vi "Save-As-Default (SubVI).vi"(0 "Current VI's Path":path, 2 "Load Settings":bool, 4 "Save Settings":bool, 9 "Save and Exit":bool) -> (19 "Save as Default Error":errorcluster)   [LabVIEW 2009]
panel:
  # "Save As Defaults (SubVI) - Created by Blake Otting - October 2007\nUpdated 4/7/2010"
  # "Connect As Shown \nin Main Program VI"
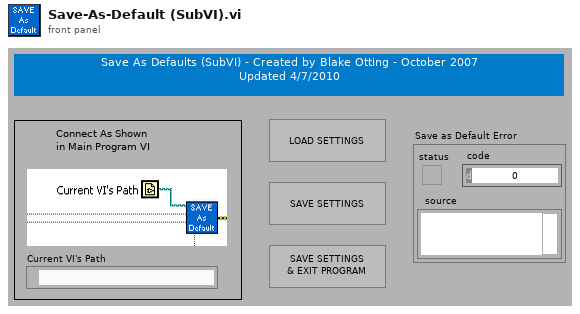
[diagram p1: front panel]
types:
  T1 = enum16{"open", "replace", "create", "open or create", "replace or create", "replace or create with confirmation"}
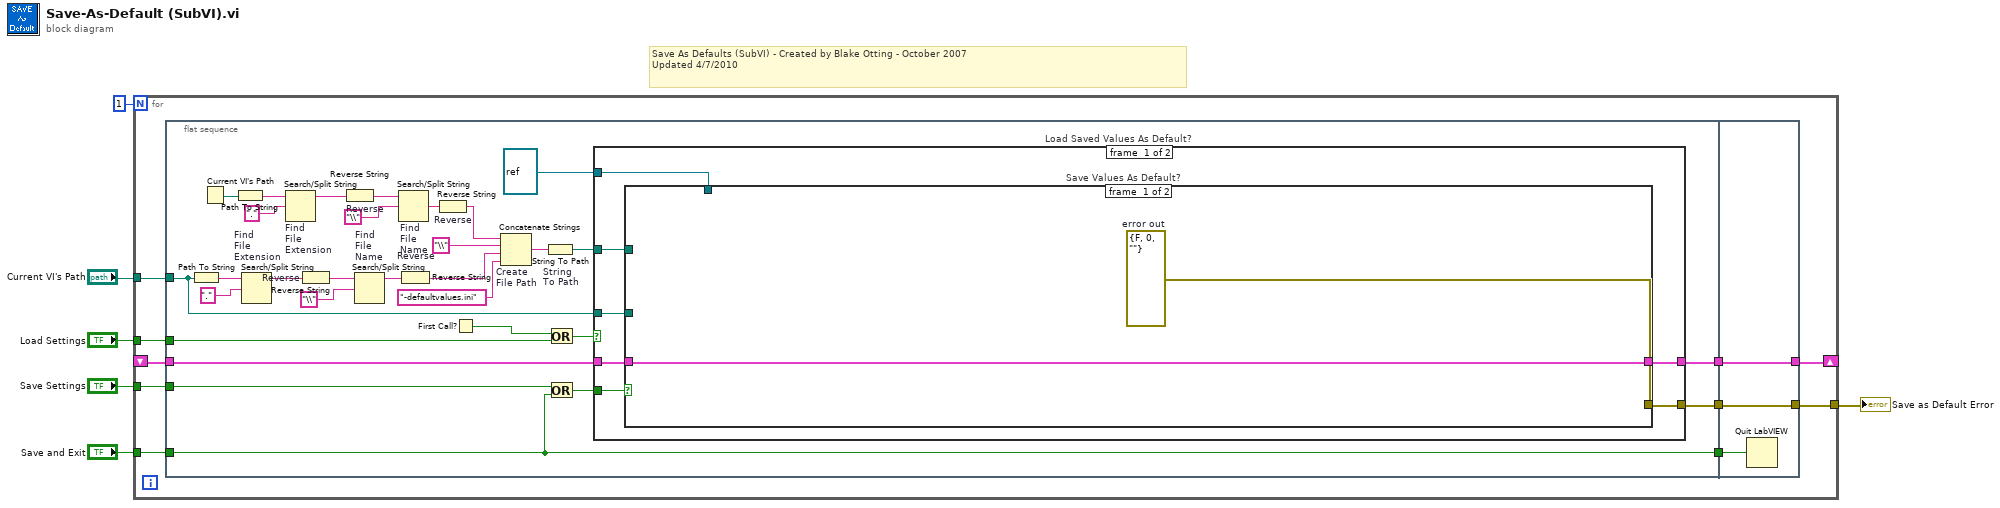
[diagram p0: block diagram]
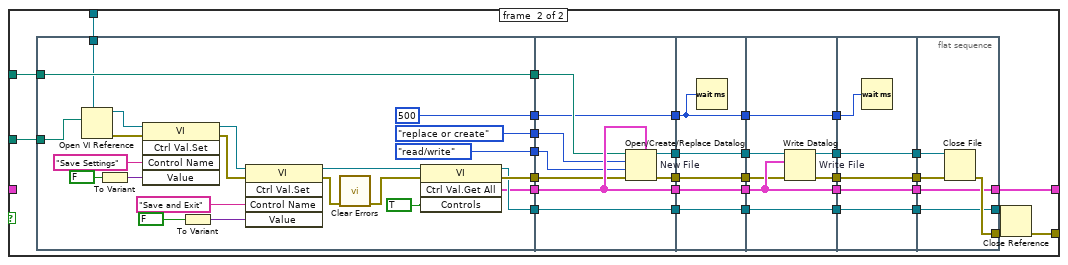
[diagram p2: hidden frame]
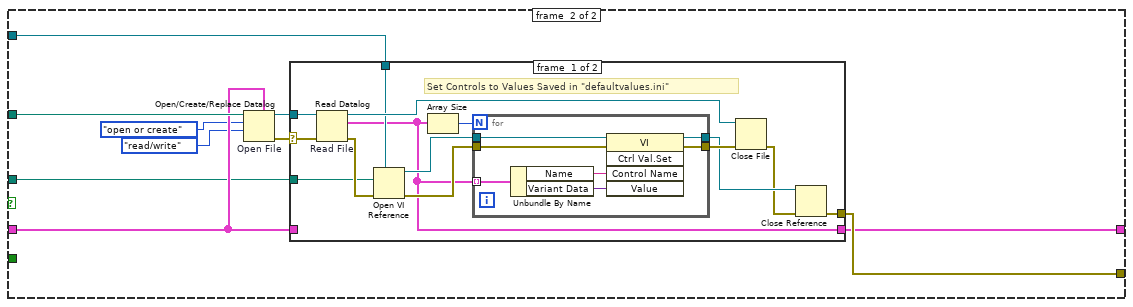
[diagram p3: hidden frame]
diagram:
  # "Save As Defaults (SubVI) - Created by Blake Otting - October 2007\nUpdated 4/7/2010"
  n1 = for {
    N: 1 -> [_]
    tunnel: "Current VI's Path" -> [w15]
    shift-right: [w16] -> _
    shift-left: _ -> [w14]
    tunnel: [w13] -> w1
    tunnel: "Save and Exit" -> [w8]
    tunnel: "Load Settings" -> [w7]
    tunnel: "Save Settings" -> [w9]
    n2 = flat-sequence {
      tunnel: [w45] -> w12
      tunnel: [w42] -> w11
      tunnel: [w41] -> w10
      tunnel: w7 -> [w39]
      tunnel: w8 -> [w41]
      tunnel: w9 -> [w40]
      tunnel: w15 -> [w38]
      tunnel: w14 -> [w46]
      tunnel: [w177] -> w13
      tunnel: [w178] -> w16
      tunnel: w12 -> [w178]
      tunnel: w11 -> [w177]
      tunnel: w10 -> [w176]
      frame #0 {
        n3 = Path To String(path=w38) -> (string=w25:string)
        n4 = Current VI's Path() -> (path=w20:path)
        n5 = Path To String(path=w20) -> (string=w32:string)
        n6 = Search/Split String "Find\nFile \nExtension"(string=w25, search string/char (-)=".") -> (substring before match=w22:string)  [unwired: 1 in, 2 out]
        n7 = Search/Split String "Find\nFile \nExtension"(string=w32, search string/char (-)=".") -> (substring before match=w31:string)  [unwired: 1 in, 2 out]
        n8 = Reverse String "Reverse"(1:w22) -> (0:w24:string)
        n9 = Reverse String "Reverse"(1:w31) -> (0:w30:string)
        n10 = Search/Split String "Find\nFile \nName"(string=w24, search string/char (-)="\\") -> (substring before match=w21:string)  [unwired: 1 in, 2 out]
        n11 = Search/Split String "Find\nFile \nName"(string=w30, search string/char (-)="\\") -> (match + rest of string=w28:string)  [unwired: 1 in, 2 out]
        n12 = Reverse String "Reverse"(1:w21) -> (0:w18:string)
        n13 = Reverse String "Reverse"(1:w28) -> (0:w27:string)
        n14 = First Call?() -> (First Call?: T/F=w34:bool)
        n15 = Concatenate Strings "Create\nFile Path"(w27, "\\", w18, "-defaultvalues.ini") -> (w36:string)
        n16 = String To Path "String\nTo Path"(string=w36) -> (path=w37:path)
        n17 = Or(x=w34, y=w39) -> (x .or. y?=w44:bool)
        n18 = Or(x=w40, y=w41) -> (x .or. y?=w43:bool)
        n19 = case "Load Saved Values As Default?" shown="False" w44 {
          tunnel: [w53 w152] -> w42
          tunnel: w37 -> [w52 w150]
          tunnel: w43 -> [w51 _]
          tunnel: w46 -> [w50 w149]
          tunnel: [w47 w151] -> w45
          tunnel: w38 -> [w49 w147]
          tunnel: refnum<vi> refnum ("Application Reference Input 2") -> [w48 w148]
          frame #0 {
            n20 = case "Save Values As Default?" shown="True" w51 {
              tunnel: [w54 w88] -> w53
              tunnel: w52 -> [_ w87]
              tunnel: [w55 w86] -> w47
              tunnel: w50 -> [w55 _]
              tunnel: w49 -> [_ w56]
              tunnel: w48 -> [_ w57]
              frame #0 {
                w54 = errorcluster {"status"=FALSE, "code"=0, "source"=""}  # error out
              }
              frame #1 {
                n21 = flat-sequence {
                  tunnel: w87 -> [w111]
                  tunnel: [w93] -> w66
                  tunnel: [enum16{"read/write", "read-only", "write-only"}."read/write" ("access (0:read/write)")] -> w65
                  tunnel: [T1."replace or create" ("operation (0:open)")] -> w64
                  tunnel: [w91] -> w63
                  tunnel: [w111] -> w62
                  tunnel: [w92] -> w61
                  tunnel: [u32 500 ("milliseconds to wait")] -> w60
                  tunnel: w57 -> [w95]
                  tunnel: w56 -> [w94]
                  tunnel: [w116] -> w85
                  tunnel: [w115] -> w83
                  tunnel: [w120] -> w81
                  tunnel: [w113] -> w79
                  tunnel: [w112] -> w67
                  tunnel: w66 -> [w119]
                  tunnel: w65 -> [w118]
                  tunnel: w64 -> [w117]
                  tunnel: w63 -> [w120]
                  tunnel: w62 -> [w114]
                  tunnel: w61 -> [w113]
                  tunnel: w60 -> [w112]
                  tunnel: w85 -> [w125]
                  tunnel: [w125] -> w84
                  tunnel: w83 -> [w124]
                  tunnel: [w124] -> w82
                  tunnel: w81 -> [w123]
                  tunnel: [w123] -> w80
                  tunnel: w79 -> [w122]
                  tunnel: [w122] -> w78
                  tunnel: w67 -> [w121]
                  tunnel: [w121] -> w58
                  tunnel: w84 -> [w130]
                  tunnel: w82 -> [w132]
                  tunnel: w80 -> [w131]
                  tunnel: [w131] -> w77
                  tunnel: w78 -> [w129]
                  tunnel: [w129] -> w75
                  tunnel: [w128] -> w73
                  tunnel: [w127] -> w71
                  tunnel: [w126] -> w59
                  tunnel: w58 -> [w126]
                  tunnel: w77 -> [w137]
                  tunnel: [w137] -> w76
                  tunnel: w75 -> [w136]
                  tunnel: [w136] -> w74
                  tunnel: w73 -> [w135]
                  tunnel: [w135] -> w72
                  tunnel: w71 -> [w134]
                  tunnel: [w134] -> w70
                  tunnel: w59 -> [w133]
                  tunnel: [w141] -> w86
                  tunnel: w76 -> [w141]
                  tunnel: [w140] -> w68
                  tunnel: w74 -> [w140]
                  tunnel: w72 -> [w139]
                  tunnel: w70 -> [w138]
                  tunnel: [w142] -> w69
                  frame #0 {
                    n22 = Open VI Reference(type specifier VI Refnum (for type only)=w95, vi path=w94) -> (vi reference=w103:refnum<vi>, error out=w104:errorcluster)  [unwired: 2 in, 2 out]
                    n23 = To Variant(anything=FALSE ("Controls")) -> (Variant=w102:variant)
                    n24 = invoke class="VI" method="Ctrl Val.Set"(reference=w103, error in=w104, "Control Name"="Save Settings", "Value"=w102) -> (reference out=w107:refnum<vi>, error out=w108:errorcluster)  [unwired: 1 in, 3 out]
                    n25 = To Variant(anything=FALSE ("Controls")) -> (Variant=w105:variant)
                    n26 = invoke class="VI" method="Ctrl Val.Set"(reference=w107, error in=w108, "Control Name"="Save and Exit", "Value"=w105) -> (reference out=w110:refnum<vi>, error out=w90:errorcluster)  [unwired: 1 in, 3 out]
                    n27 = call <vilib>:"Clear Errors.vi"("error in (no error)"=w90) -> ("error out"=w89:errorcluster)  [unwired: 6 out]
                    n28 = invoke class="VI" method="Ctrl Val.Get All"(reference=w110, error in=w89, "Controls"=TRUE) -> (reference out=w92:refnum<vi>, error out=w93:errorcluster, "Get All Control Values Variant"=w91:cluster{"Name":string, "Variant Data":variant}[])  [unwired: 1 in, 1 out]
                  }
                  frame #1 {
                    n29 = Open/Create/Replace Datalog "New File"(5:w120, 8:w119, 9:w118, 10:w117, 11:w114) -> (0:w116:errorcluster, 3:w115:refnum<k1>)  [unwired: 2 out]
                  }
                  frame #2 {
                    n30 = Wait (ms)(milliseconds to wait=w121) -> ()  [unwired: 1 out]
                  }
                  frame #3 {
                    n31 = Write Datalog "Write File"(4:w130, 6:w131, 7:w132) -> (0:w128:errorcluster, 3:w127:refnum<k1>)
                  }
                  frame #4 {
                    n32 = Wait (ms)(milliseconds to wait=w133) -> ()  [unwired: 1 out]
                  }
                  frame #5 {
                    n33 = Close File(refnum=w138, error in=w139) -> (error out=w142:errorcluster)  [unwired: 1 out]
                  }
                }
                n34 = Close Reference(reference=w68, error in (no error)=w69) -> (error out=w88:errorcluster)
              }
            }
          }
          frame #1 {
            n35 = Open/Create/Replace Datalog "Open File"(5:w149, 9:enum16{"read/write", "read-only", "write-only"}."read/write" ("access (0:read/write)"), 10:T1."open or create" ("operation (0:open)"), 11:w150) -> (0:w146:errorcluster, 3:w145:refnum<k1>)  [unwired: 1 in, 2 out]
            n36 = case shown="No Error" w146 {
              selector: w146 -> [w160 w174]
              tunnel: [w164 w174] -> w152
              tunnel: w149 -> [_ w175]
              tunnel: [w153 w175] -> w151
              tunnel: w145 -> [w161 _]
              tunnel: w148 -> [w157 _]
              tunnel: w147 -> [w156 _]
              frame #0 {
                # "Set Controls to Values Saved in \"defaultvalues.ini\""
                n37 = Read Datalog "Read File"(4:w160, 7:w161) -> (0:w158:errorcluster, 2:w153:cluster{"Name":string, "Variant Data":variant}[], 3:w166:refnum<k1>)  [unwired: 1 out]
                n38 = Open VI Reference(type specifier VI Refnum (for type only)=w157, vi path=w156, error in (no error)=w158) -> (vi reference=w159:refnum<vi>, error out=w155:errorcluster)  [unwired: 1 in, 2 out]
                n39 = Array Size(array=w153) -> (size(s)=w154:i32)
                n40 = for {
                  N: w154 -> [_]
                  tunnel: w153 -> [w169] mode=indexing
                  tunnel: w155 -> [w171]
                  tunnel: [w172] -> w165
                  tunnel: w159 -> [w170]
                  tunnel: [w167] -> w163
                  n41 = Unbundle By Name(w169) -> ("Name"=w168:string, "Variant Data"=w173:variant)
                  n42 = invoke class="VI" method="Ctrl Val.Set"(reference=w170, error in=w171, "Control Name"=w168, "Value"=w173) -> (reference out=w167:refnum<vi>, error out=w172:errorcluster)  [unwired: 1 in, 3 out]
                }
                n43 = Close File(refnum=w166, error in=w165) -> (error out=w162:errorcluster)  [unwired: 1 out]
                n44 = Close Reference(reference=w163, error in (no error)=w162) -> (error out=w164:errorcluster)
              }
              frame #1 {
                # "\"defaultvalues.ini\" Not Found"
              }
            }
          }
        }
      }
      frame #1 {
        n45 = Quit LabVIEW(quit? (T)=w176) -> ()
      }
    }
  }
  "Save as Default Error" <- w1
